vi "Do.vi"(8 "error in (no error)":errorcluster, 10 "Actor in":refnum<class "Actor.lvclass">, 11 "Configure Channel Msg":refnum<class "Configure Channel Msg.lvclass">) -> (0 "error out":errorcluster, 2 "Actor out":refnum<class "Actor.lvclass">)   [LabVIEW 2015, in "CS++Scope.lvlib" / "Configure Channel Msg.lvclass"]
doc: "This VI delivers the message to the actor by calling the appropriate method(s) on the actor."
uses:
  Configure Channel Msg.lvclass
  CS++Scope/CS++Scope.lvclass
  CSPP_Core/Actors/CS++PVMonitor Messages/CS++PVUpdate Msg/CS++PVUpdate Msg.lvclass
  CSPP_Core/Classes/CS++ProcessVariables/ProcessVariable/PV.lvclass
  <vilib>/ActorFramework/Actor/Actor.lvclass
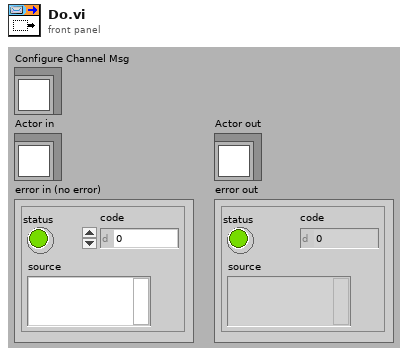
[diagram p1: front panel]
types:
  T1 = cluster{"channel enabled (True)":bool, "channel name (\"CHANNEL1\")":string, "probe attenuation (1:1.0)":dbl, "vertical offset (0.0 V)":dbl[unit], "vertical coupling (DC)":i32, "vertical range (10.0 V)":dbl[unit]}
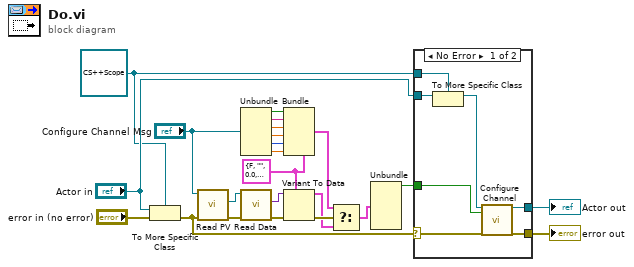
[diagram p0: block diagram]
diagram:
  w15 = T1 {"channel enabled (True)"=FALSE, "channel name (\"CHANNEL1\")"="", "probe attenuation (1:1.0)"=0.0, "vertical offset (0.0 V)"=0.0, "vertical coupling (DC)"=0, "vertical range (10.0 V)"=0.0} ("Type")
  w19 = refnum<class "CS++Scope.lvclass"> refnum ("Actor in")
  n1 = To More Specific Class(target class=w19, reference="Actor in", error in="error in (no error)") -> (error out=w8:errorcluster)  [unwired: 1 out]
  n2 = call "Read PV.vi"("error in (no error)"=w8, "CS++PVUpdate Msg in"="Configure Channel Msg") -> ("error out"=w18:errorcluster, "PV"=w14:refnum<class "PV.lvclass">)  [unwired: 7 in, 1 out]
  n3 = Unbundle ("Pre-Unbundler")("Configure Channel Msg") -> (w6:bool, w5:string, w4:dbl, w3:dbl[unit], w2:i32, w1:dbl[unit])
  n4 = call "Read Data.vi"("error in (no error)"=w18, "PV in"=w14) -> ("error out"=w12:errorcluster, "Data"=w13:variant)  [unwired: 7 in, 1 out]
  n5 = Bundle ("Pre-Bundler")(cluster=w15, "channel enabled (True)"=w6, "channel name (\"CHANNEL1\")"=w5, "probe attenuation (1:1.0)"=w4, "vertical offset (0.0 V)"=w3, "vertical coupling (DC)"=w2, "vertical range (10.0 V)"=w1) -> (w16:T1)
  n6 = Variant To Data(error in=w12, type=w15, Variant=w13) -> (data=w10:T1, error out=w17:errorcluster)
  n7 = Select ("MainSelect")(t=w16, s=w17, f=w10) -> (s? t:f=w11:T1)
  n8 = Unbundle ("Main-Unbundler")(w11) -> ("channel enabled (True)"=w7:bool)  [unwired: 5 out]
  n9 = case shown="No Error" w8 {
    selector: w8 -> [w28 w32]
    tunnel: [w30 w32] -> w22
    tunnel: [w29 w31] -> w21
    tunnel: "Actor in" -> [w27 w31]
    tunnel: w19 -> [w26 _]
    tunnel: w7 -> [w24 _]
    frame No Error {
      n10 = To More Specific Class(target class=w26, reference=w27) -> (specific class reference=w25:refnum<class "CS++Scope.lvclass">)  [unwired: 1 in, 1 out]
      n11 = call "Configure Channel.vi"("CS++Scope"=w25, "channel enabled (True)"=w24, "error in (no error)"=w28) -> ("CS++Scope out"=w29:refnum<class "CS++Scope.lvclass">, "error out"=w30:errorcluster)  [unwired: 15 in]
    }
    frame Error {
    }
  }
  "error out" <- w22
  "Actor out" <- w21
